vi "Get Configurations.vi"(11 "Component in":refnum<class "Component.lvclass">) -> (2 "Configurations":refnum<class "Component Configurations.lvclass">, 3 "Component out":refnum<class "Component.lvclass">)   [LabVIEW 2019, in "DSF Core.lvlib" / "Component.lvclass"]
uses:
  Component.lvclass
  Component Configuration/Component Configurations.lvclass
  Component.lvclass/Component.ctl
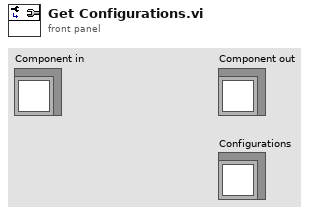
[diagram p1: front panel]
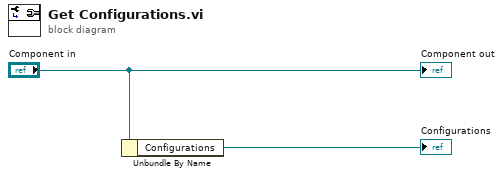
[diagram p0: block diagram]
diagram:
  n1 = Unbundle By Name("Component in") -> ("Configurations"=→"Configurations":refnum<class "Component Configurations.lvclass">)
  "Component out" <- "Component in"
